vi "test - timestamp.vi"(8 "error in (no error)":errorcluster, 11 "TestCase in":refnum<class "testcase-Supported-Datatype.lvclass">) -> (0 "error out":errorcluster, 3 "TestCase out":refnum<class "testcase-Supported-Datatype.lvclass">)   [LabVIEW 2017, in "testcase-Supported-Datatype.lvclass"]
uses:
  testcase-Supported-Datatype.lvclass
  <vilib>/addons/_JKI Toolkits/VI Tester/TestCase.llb/TestCase.lvclass
  addons/API-String-Arugments-Support/API String Arguments Support.lvlib
  C:/Program Files (x86)/National Instruments/LabVIEW 2017/vi.lib/addons/_JKI Toolkits/VI Tester/TestCase.llb/TestCase.lvclass
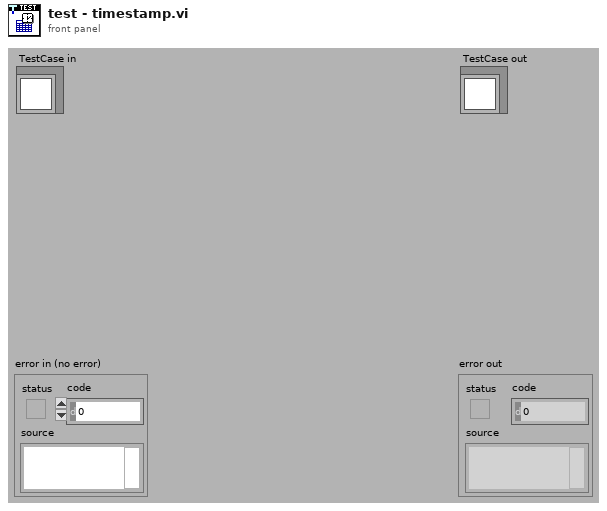
[diagram p1: front panel]
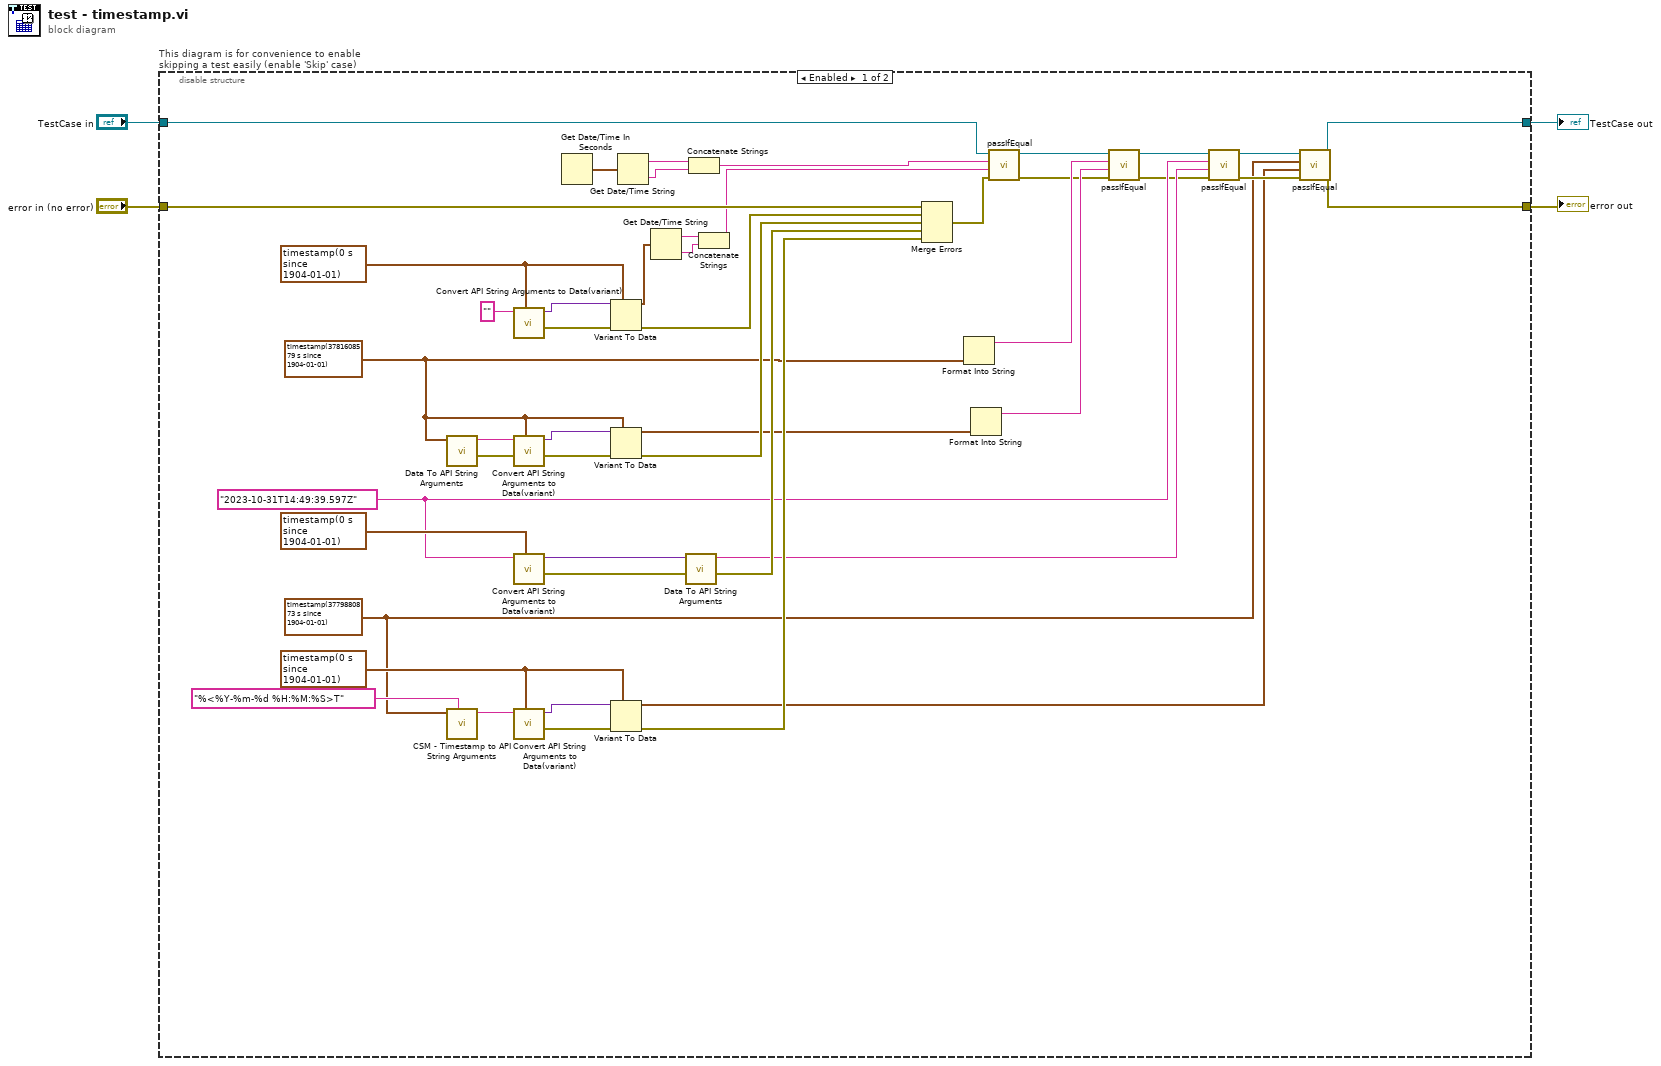
[diagram p0: block diagram]
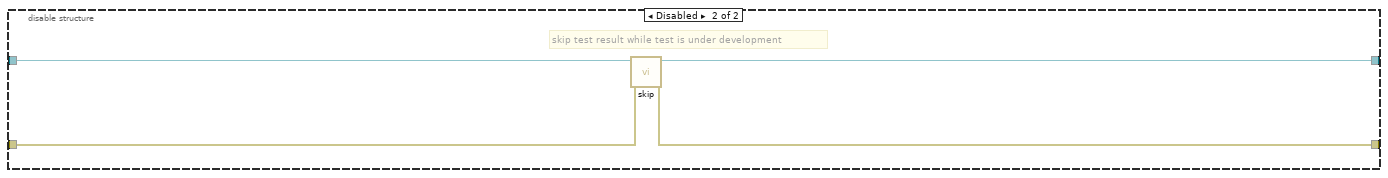
[diagram p2: hidden frame]
diagram:
  n1 = disable-structure "This diagram is for convenience to enable skipping a test easily (enable 'Skip' case)" shown="Enabled" {
    disable-tunnel: "TestCase in" -> [w14 w55]
    disable-tunnel: [w25 w53] -> w1
    disable-tunnel: [w26 w54] -> w3
    disable-tunnel: "error in (no error)" -> [w22 w52]
    frame Enabled {
      w24 = timestamp(3779880873 s since 1904-01-01) ("Time Stamp 3")
      w32 = "2023-10-31T14:49:39.597Z" ("String")
      w19 = timestamp(3781608579.597416 s since 1904-01-01) ("Time Stamp 1")
      w41 = timestamp(0 s since 1904-01-01) ("Time Stamp")
      w46 = timestamp(0 s since 1904-01-01) ("Time Stamp")
      n2 = call "Data To API String Arguments.vi"("data"=w19) -> ("error out"=w50:errorcluster, "String"=w51:string)  [unwired: 9 in]
      n3 = call "CSM - Timestamp to API String Arguments.vi"("Format (Empty to Use UTC)"="%<%Y-%m-%d %H:%M:%S>T" ("format string"), "Timestamp (now)"=w24) -> ("API String"=w33:string)  [unwired: 8 in, 1 out]
      n4 = call "Convert API String Arguments to Data(variant).vi"("Type"=w41, "String"="" ("Empty String")) -> ("error"=w39:errorcluster, "Data"=w40:variant)  [unwired: 8 in]
      n5 = call "Convert API String Arguments to Data(variant).vi"("Type"=w19, "error in (no error)"=w50, "String"=w51) -> ("error"=w49:errorcluster, "Data"=w43:variant)  [unwired: 7 in]
      n6 = call "Convert API String Arguments to Data(variant).vi"("Type"=timestamp(0 s since 1904-01-01) ("Time Stamp"), "String"=w32) -> ("error"=w48:errorcluster, "Data"=w21:variant)  [unwired: 8 in]
      n7 = call "Convert API String Arguments to Data(variant).vi"("Type"=w46, "String"=w33) -> ("error"=w47:errorcluster, "Data"=w45:variant)  [unwired: 8 in]
      n8 = Get Date/Time In Seconds() -> (seconds since 1Jan1904=w11:timestamp)
      n9 = Variant To Data(error in=w39, type=w41, Variant=w40) -> (data=w10:timestamp, error out=w37:errorcluster)
      n10 = Variant To Data(error in=w49, type=w19, Variant=w43) -> (data=w20:timestamp, error out=w36:errorcluster)
      n11 = Variant To Data(error in=w47, type=w46, Variant=w45) -> (data=w23:timestamp, error out=w34:errorcluster)
      n12 = Get Date/Time String(seconds (now)=w11) -> (date string=w12:string, time string=w8:string)  [unwired: 2 in]
      n13 = Get Date/Time String(seconds (now)=w10) -> (date string=w7:string, time string=w6:string)  [unwired: 2 in]
      n14 = call "Data To API String Arguments.vi"("error in (no error)"=w48, "data"=w21) -> ("error out"=w35:errorcluster, "String"=w31:string)  [unwired: 8 in]
      n15 = Concatenate Strings(w12, w8) -> (w9:string)
      n16 = Concatenate Strings(w7, w6) -> (w5:string)
      n17 = Merge Errors(w22, w37, w36, w35, w34) -> (w15:errorcluster)
      n18 = Format Into String(w19) -> (resulting string=w18:string)  [unwired: 3 in, 1 out]
      n19 = Format Into String(w20) -> (resulting string=w17:string)  [unwired: 3 in, 1 out]
      n20 = call-dynamic "passIfEqual.vi"("error in (no error)"=w15, "y"=w5, "x"=w9, "TestCase in"=w14) -> ("error out"=w16:errorcluster, "TestCase out"=w13:refnum<class "testcase-Supported-Datatype.lvclass">)  [unwired: 6 in]
      n21 = call-dynamic "passIfEqual.vi"("error in (no error)"=w16, "y"=w17, "x"=w18, "TestCase in"=w13) -> ("error out"=w30:errorcluster, "TestCase out"=w29:refnum<class "testcase-Supported-Datatype.lvclass">)  [unwired: 6 in]
      n22 = call-dynamic "passIfEqual.vi"("error in (no error)"=w30, "y"=w31, "x"=w32, "TestCase in"=w29) -> ("error out"=w27:errorcluster, "TestCase out"=w28:refnum<class "testcase-Supported-Datatype.lvclass">)  [unwired: 6 in]
      n23 = call-dynamic "passIfEqual.vi"("error in (no error)"=w27, "y"=w23, "x"=w24, "TestCase in"=w28) -> ("error out"=w26:errorcluster, "TestCase out"=w25:refnum<class "testcase-Supported-Datatype.lvclass">)  [unwired: 6 in]
    }
    frame Disabled {
      # "skip test result while test is under development"
      n24 = call <vilib>:"skip.vi"("error in (no error)"=w52, "TestCase in"=w55) -> ("error out"=w54:errorcluster, "TestCase out"=w53:refnum<class "testcase-Supported-Datatype.lvclass">)  [unwired: 8 in]
    }
  }
  "error out" <- w3
  "TestCase out" <- w1
